vi "cal.vi"(0 "Step1":string[](array[string]), 1 "Step3":string[](array[string]), 2 "Step4":string[](array[string]), 3 "x 固定距离":dbl=2.355000000000018, 4 "y固定距离":dbl=1137.7340000000002, 5 "分辨率":dbl=0.0045 format="%#_13g", 6 "Point1 (Pixels)":cluster{"X":sgl, "Y":sgl}, 7 "Angle (Real-World)":dbl, 8 "Point2 (Pixels)":cluster{"X":sgl, "Y":sgl}) -> (13 "数值":dbl, 14 "Y 距离 同屏幕":dbl[](array[numeric]), 16 "X 距离 同屏幕":dbl[](array[numeric]), 19 "计算角度":dbl)   [LabVIEW 2015]
uses:
  <vilib>/vision/NI_Vision_Development_Module.lvlib
  <vilib>/Analysis/NI_AALPro.lvlib
panel:
  out "添加的数组":cluster{"X":sgl, "Y":sgl}[](array[cluster])
  out "Distances":sgl[](array[numeric]) format="%.4f"
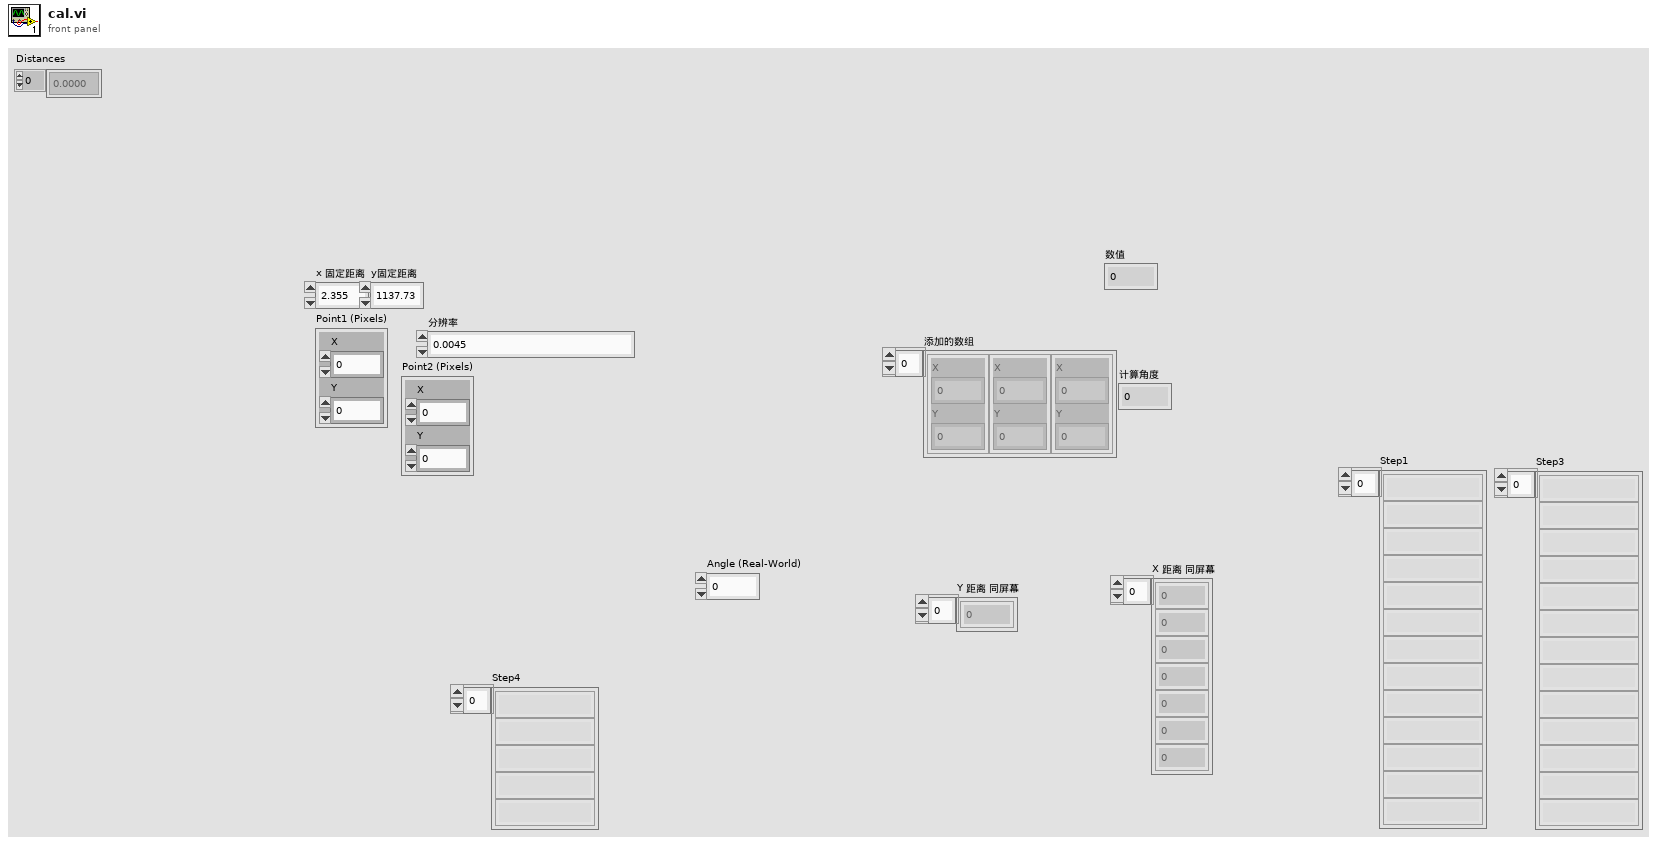
[diagram p1: front panel]
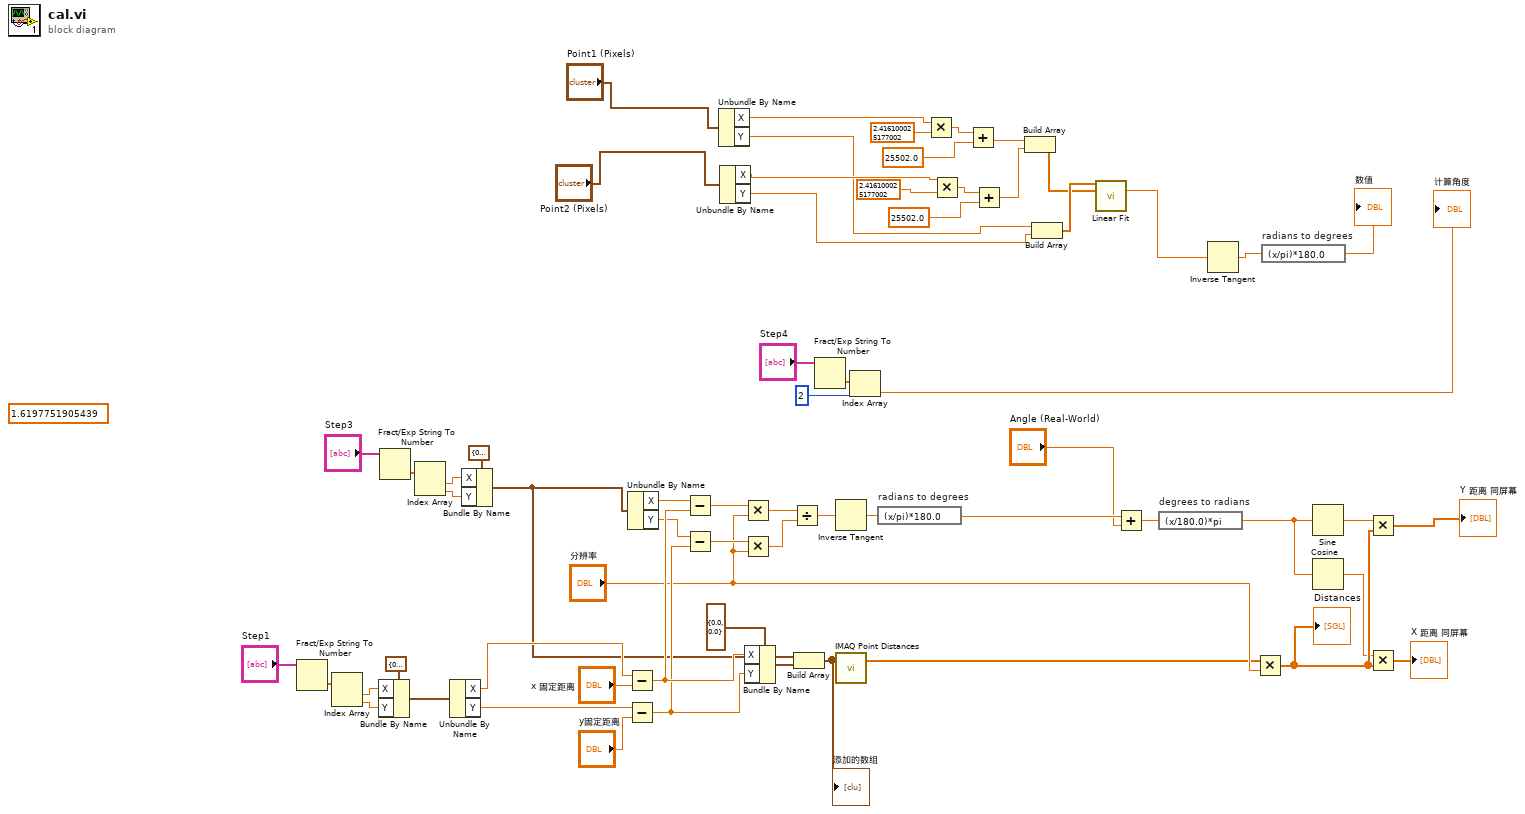
[diagram p0: block diagram]
diagram:
  (unwired) 1.6197751905439 ("x")
  n1 = Fract/Exp String To Number(string="Step1") -> (number=w27:dbl[])  [unwired: 3 in, 1 out]
  n2 = Index Array(array=w27) -> (element #1=w29:dbl, element #2=w30:dbl)  [unwired: 2 in]
  n3 = Bundle By Name(cluster=cluster{"X":sgl, "Y":sgl} {"X"=0.0, "Y"=0.0} ("Center (Pixels)"), "X"=w29, "Y"=w30) -> (w25:cluster{"X":sgl, "Y":sgl})
  n4 = Fract/Exp String To Number(string="Step3") -> (number=w35:dbl[])  [unwired: 3 in, 1 out]
  n5 = Index Array(array=w35) -> (element #1=w33:dbl, element #2=w32:dbl)  [unwired: 2 in]
  n6 = Unbundle By Name(w25) -> ("X"=w59:sgl, "Y"=w58:sgl)
  n7 = Bundle By Name(cluster=cluster{"X":sgl, "Y":sgl} {"X"=0.0, "Y"=0.0} ("Center (Pixels)"), "X"=w33, "Y"=w32) -> (w31:cluster{"X":sgl, "Y":sgl})
  n8 = Subtract(x=w59, y="x 固定距离") -> (x-y=w55:dbl)
  n9 = Subtract(x=w58, y="y固定距离") -> (x-y=w53:dbl)
  n10 = Unbundle By Name(w31) -> ("X"=w56:sgl, "Y"=w54:sgl)
  n11 = Subtract(x=w56, y=w55) -> (x-y=w61:dbl)
  n12 = Subtract(x=w54, y=w53) -> (x-y=w60:dbl)
  n13 = Unbundle By Name("Point1 (Pixels)") -> ("X"=w13:sgl, "Y"=w9:sgl)
  n14 = Unbundle By Name("Point2 (Pixels)") -> ("X"=w12:sgl, "Y"=w8:sgl)
  n15 = Multiply(x=w61, y="分辨率") -> (x*y=w52:dbl)
  n16 = Multiply(x=w60, y="分辨率") -> (x*y=w51:dbl)
  n17 = Bundle By Name(cluster=cluster{"X":sgl, "Y":sgl} {"X"=0.0, "Y"=0.0} ("Center (Pixels)1 4"), "X"=w55, "Y"=w53) -> (w48:cluster{"X":sgl, "Y":sgl})
  n18 = Divide(x=w52, y=w51) -> (x/y=w49:dbl)
  n19 = Build Array(w31, w48) -> (w47:cluster{"X":sgl, "Y":sgl}[])
  "添加的数组" <- w47
  n20 = Fract/Exp String To Number(string="Step4") -> (number=w24:dbl[])  [unwired: 3 in, 1 out]
  n21 = Inverse Tangent(1:w49) -> (0:w50:dbl)
  n22 = call "IMAQ Point Distances"("Points"=w47) -> ("Distances"=w45:sgl[])  [unwired: 4 in, 1 out]
  n23 = Index Array(array=w24, index=2 ("索引")) -> (element=→"计算角度":dbl)
  n24 = expression code="(x/pi)*180.0" "radians to degrees"(w50) -> (w44:dbl)
  n25 = Multiply(x=w13, y=sgl 2.4161) -> (x*y=w18:sgl)
  n26 = Multiply(x=w12, y=sgl 2.4161) -> (x*y=w15:sgl)
  n27 = Add(x=w18, y=sgl 25502.0) -> (x+y=w10:sgl)
  n28 = Add(x=w15, y=sgl 25502.0) -> (x+y=w11:sgl)
  n29 = Build Array(w10, w11) -> (w4:sgl[])
  n30 = Build Array(w9, w8) -> (w5:sgl[])
  n31 = call <vilib>:"Linear Fit.vi"("Y"=w5, "X"=w4) -> ("slope"=w20:dbl)  [unwired: 9 in, 4 out]
  n32 = Add(x=w44, y="Angle (Real-World)") -> (x+y=w43:dbl)
  n33 = expression code="(x/180.0)*pi" "degrees to radians"(w43) -> (w40:dbl)
  n34 = Inverse Tangent(1:w20) -> (0:w21:dbl)
  n35 = Multiply(x=w45, y="分辨率") -> (x*y=w39:dbl[])
  "Distances" <- w39
  n36 = expression code="(x/pi)*180.0" "radians to degrees"(w21) -> (→"数值":dbl)
  n37 = Sine(x=w40) -> (sin(x)=w41:dbl)
  n38 = Cosine(x=w40) -> (cos(x)=w38:dbl)
  n39 = Multiply(x=w41, y=w39) -> (x*y=→"Y 距离 同屏幕":dbl[])
  n40 = Multiply(x=w38, y=w39) -> (x*y=→"X 距离 同屏幕":dbl[])
